vi "Write Disabled.vi"(8 "error in (no error)":errorcluster, 10 "Disabled":T1(ring), 11 "Reference Control in":refnum<class "Reference Control.lvclass">) -> (0 "error out":errorcluster, 3 "Reference Control out":refnum<class "Reference Control.lvclass">)   [LabVIEW 2016, in "Reference Control.lvclass"]
uses:
  Reference Control.lvclass
  Reference Control.lvclass/Reference Control.ctl
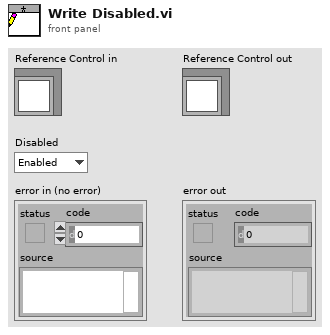
[diagram p1: front panel]
types:
  T1 = enum8{"Enabled", "Disabled", "Disabled and Grayed Out"}
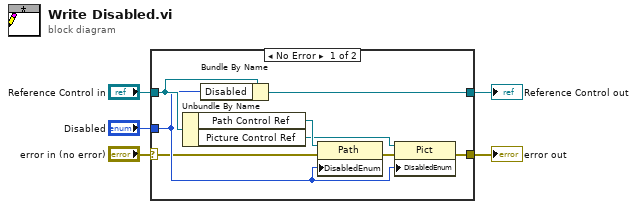
[diagram p0: block diagram]
diagram:
  n1 = case shown="No Error" "error in (no error)" {
    selector: "error in (no error)" -> [w8 w14]
    tunnel: [w6 w14] -> w4
    tunnel: [w13 w15] -> w2
    tunnel: "Reference Control in" -> [w12 w15]
    tunnel: "Disabled" -> [w9 _]
    frame No Error {
      n2 = Unbundle By Name(w12) -> ("Path Control Ref"=w11:refnum<vi>, "Picture Control Ref"=w10:refnum<vi>)
      n3 = Bundle By Name(cluster=w12, "Disabled"=w9) -> (w13:refnum<class "Reference Control.lvclass">)
      n4 = property class="Path"(reference=w11, error in=w8, "DisabledEnum"=w9) -> (error out=w7:errorcluster)  [unwired: 1 out]
      n5 = property class="Pict"(reference=w10, error in=w7, "DisabledEnum"=w9) -> (error out=w6:errorcluster)  [unwired: 1 out]
    }
    frame Error {
    }
  }
  "error out" <- w4
  "Reference Control out" <- w2
